vi "Close Connection.vi"(8 "error in (no error)":errorcluster, 11 "object in":refnum<class "NXP.lvclass">) -> (0 "error out":errorcluster, 3 "object out":refnum<class "NXP.lvclass">)   [LabVIEW 2020, in "NXP.lvclass"]
doc: "Este vi de close conection, se utiliza para cerrar la comunicación de manera adecuada con el microcontrolador, de esta manera no se queda la comunicación activa y se deja el puerto habilitado"
uses:
  NXP.lvclass
  NXP.lvclass/NXP.ctl
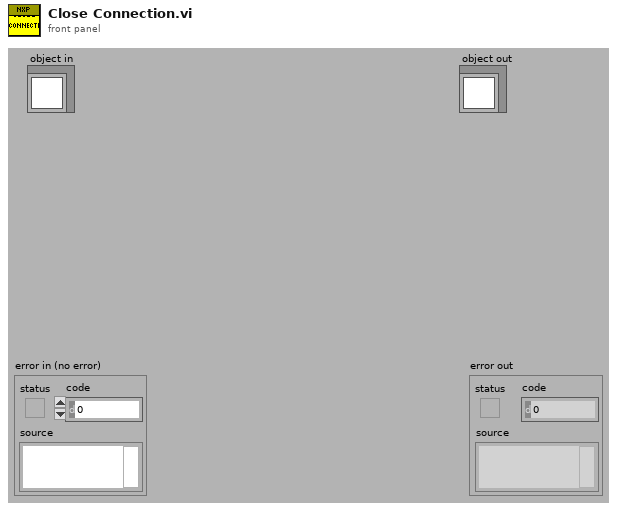
[diagram p1: front panel]
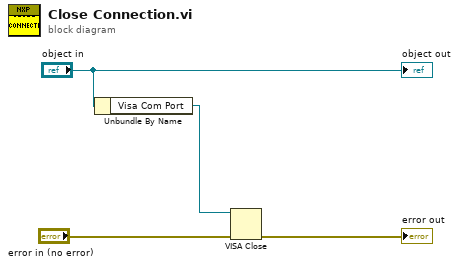
[diagram p0: block diagram]
diagram:
  n1 = Unbundle By Name("object in") -> ("Visa Com Port"=w1:refnum<visa-resource-name>)
  n2 = VISA Close(VISA resource name=w1, error in (no error)="error in (no error)") -> (error out=→"error out":errorcluster)
  "object out" <- "object in"
